vi "Generate Accuracy Report Portion.vi"(8 "error in (no error)":errorcluster, 9 "Max Accuracy %FS":dbl, 10 "Accuracy Table":string[][](array[string]), 11 "NI_report in":refnum<class "NI_report.lvclass">) -> (0 "error out":errorcluster, 3 "NI_report out":refnum<class "NI_report.lvclass">)   [LabVIEW 2026, in "Analysis.lvlib"]
uses:
  <vilib>/Utility/NIReport.llb/NI_report.lvclass
  <vilib>/Utility/NIReport.llb/Append Report Text (str wrap).vi
  <vilib>/Utility/NIReport.llb/Append Text Table to Report (wrap).vi
  Analysis.lvlib
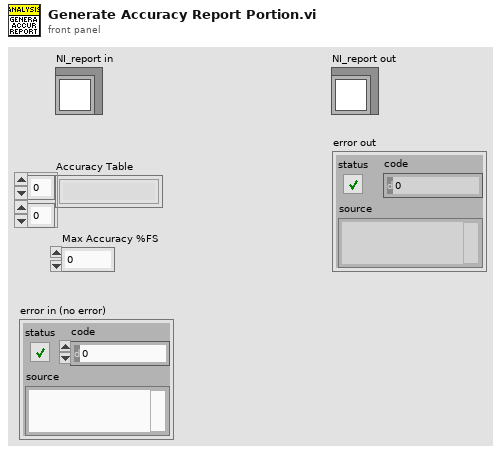
[diagram p1: front panel]
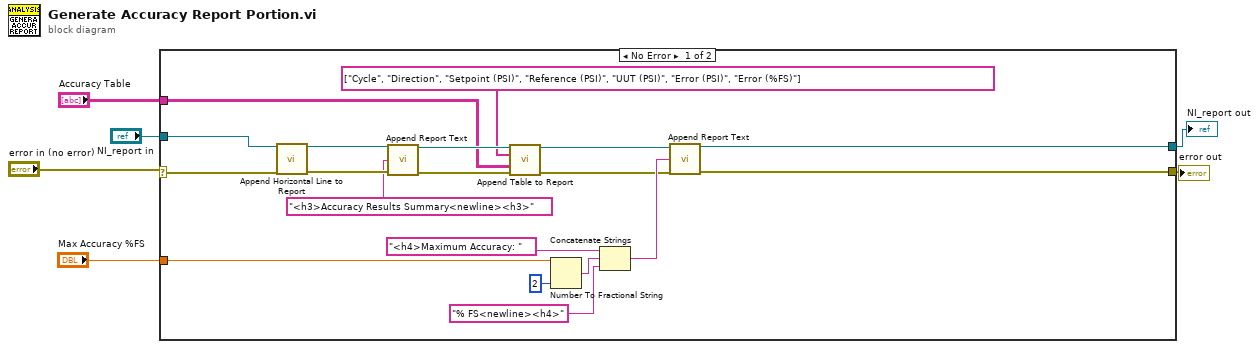
[diagram p0: block diagram]
diagram:
  n1 = case shown="No Error" "error in (no error)" {
    selector: "error in (no error)" -> [w7 w26]
    tunnel: "Max Accuracy %FS" -> [w20 _]
    tunnel: [w19 w27] -> w5
    tunnel: [w17 w26] -> w4
    tunnel: "NI_report in" -> [w13 w27]
    tunnel: "Accuracy Table" -> [w9 _]
    frame No Error {
      n2 = call-dynamic "Append Horizontal Line to Report.vi"("report in"=w13, "error in (no error)"=w7) -> ("report out"=w12:refnum<class "NI_report.lvclass">, "error out"=w11:errorcluster)  [unwired: 12 in]
      n3 = call-poly <vilib>:"Append Report Text.vi"("report in"=w12, "text"="<h3>Accuracy Results Summary<newline><h3>", "error in (no error)"=w11) -> ("report out"=w15:refnum<class "NI_report.lvclass">, "error out"=w14:errorcluster)  [unwired: 9 in, 2 out]
      n4 = call-poly <vilib>:"Append Table to Report.vi"("report in"=w15, "column headers"=string[] ["Cycle", "Direction", "Setpoint (PSI)", "Reference (PSI)", "UUT (PSI)", "Error (PSI)", "Error (%FS)"], "text data"=w9, "error in (no error)"=w14) -> ("report out"=w18:refnum<class "NI_report.lvclass">, "error out"=w16:errorcluster)  [unwired: 8 in, 2 out]
      n5 = Number To Fractional String(number=w20, precision (6)=i16 2) -> (F-format string=w22:string)  [unwired: 2 in]
      n6 = Concatenate Strings("<h4>Maximum Accuracy: ", w22, "% FS<newline><h4>") -> (w25:string)
      n7 = call-poly <vilib>:"Append Report Text.vi"("report in"=w18, "text"=w25, "error in (no error)"=w16) -> ("report out"=w19:refnum<class "NI_report.lvclass">, "error out"=w17:errorcluster)  [unwired: 9 in, 2 out]
    }
    frame Error {
    }
  }
  "NI_report out" <- w5
  "error out" <- w4
